vi "Write SP Operation Parameters.vi"(8 "error in (no error)":errorcluster, 10 "SP Operation Parameters":T1={"SP Load Less Than Thr?"=TRUE, "SP Load Threshold (um)"=4800.0, "SP Current Location"={"X (um)"=20.0, "Y (um)"=20.0, "Z (um)"=20.0, "T (degree)"=20.0}, "SP Chuck Speeds"={"XY Speed (10-100%)"=10.0, "Z Speed (10-100%)"=10.0, "T Speed (10-100%)"=10.0}, "Manual Step Parameters"={"Step in X"=FALSE, "X S-Speed [µm/step]"=5.0, "Step in Y"=FALSE, "Y S-Speed [µm/step]"=5.0, "Step in Z"=FALSE, "Z S-Speed [µm/step]"=5.0, "Step in T"=FALSE, "T S-Speed [mdegree/step]"=5.0, "X Increase"=TRUE, "Y Increase?"=TRUE, "Z Increase?"=TRUE, "T Increase?"=TRUE}, "Z Stepper"={"UP/DOWN"=FALSE, "UP/DOWN Speed [µm/step]"=20, "SP Z Step"=FALSE}, "Z Heights Set"=FALSE, "SP Contact Search"={"Contact Circuit"=enum."1", "Speed [1000-10000]"=1000.0, "Start Height [µm]"=0.0, "Search Band [µm]"=100.0, "Overdrive [µm]"=30.0}, "Separation Distance [µm]"=0, "Contact Height [µm]"=0, "Use Overdrive?"=FALSE, "Touchdown method"=enum."no feedback", "Arduino Edgesense params"={"touchdown height [µm]"=0, "search band [µm]"=100, "speed [µm/step]"=10, "overdrive [µm]"=30}} {"SP Contact Search"."Speed [1000-10000]" min=1000 max=10000; "SP Load Threshold (um)" format="%#_6f"}, 11 "SemiProbe in":refnum<class "SemiProbe.lvclass">) -> (0 "error out":errorcluster, 3 "SemiProbe out":refnum<class "SemiProbe.lvclass">)   [LabVIEW 2018, in "SemiProbe.lvclass"]
uses:
  SemiProbe.lvclass
  SemiProbe.lvclass/SemiProbe.ctl
panel:
  # "Of value set in the SP Navigation panel."
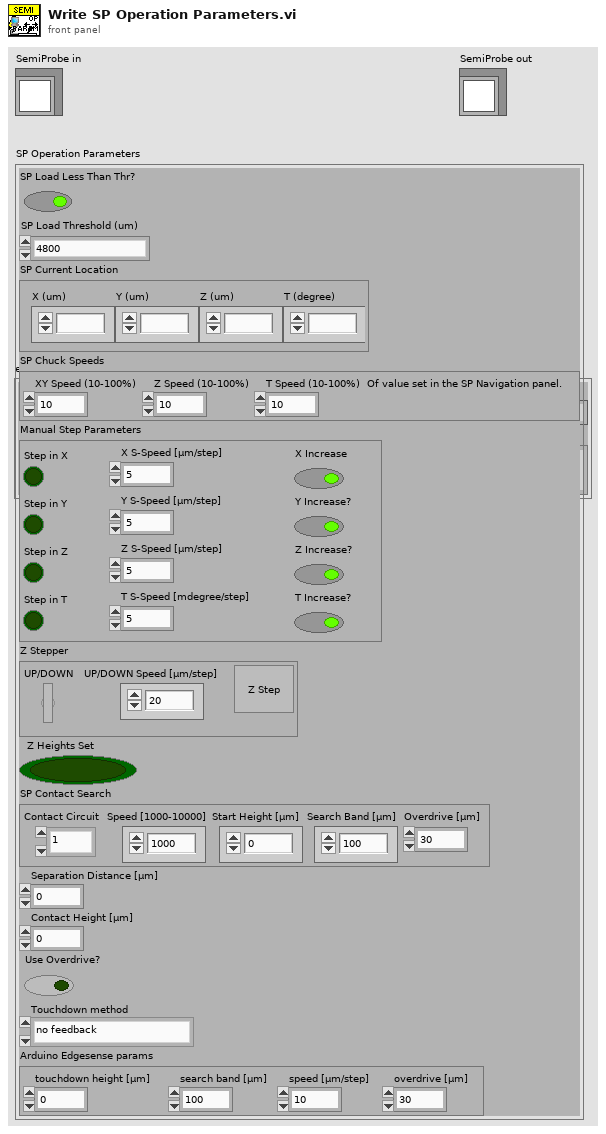
[diagram p1: front panel]
types:
  T1 = cluster{"SP Load Less Than Thr?":bool, "SP Load Threshold (um)":dbl, "SP Current Location":cluster{"X (um)":ext, "Y (um)":ext, "Z (um)":ext, "T (degree)":ext}, "SP Chuck Speeds":cluster{"XY Speed (10-100%)":dbl, "Z Speed (10-100%)":dbl, "T Speed (10-100%)":dbl}, "Manual Step Parameters":cluster{"Step in X":bool, "X S-Speed [µm/step]":sgl, "Step in Y":bool, "Y S-Speed [µm/step]":sgl, "Step in Z":bool, "Z S-Speed [µm/step]":sgl, "Step in T":bool, "T S-Speed [mdegree/step]":sgl, "X Increase":bool, "Y Increase?":bool, "Z Increase?":bool, "T Increase?":bool}, "Z Stepper":cluster{"UP/DOWN":bool, "UP/DOWN Speed [µm/step]":i32, "SP Z Step":bool}, "Z Heights Set":bool, "SP Contact Search":cluster{"Contact Circuit":enum16{"12", "1", "2"}, "Speed [1000-10000]":sgl, "Start Height [µm]":sgl, "Search Band [µm]":sgl, "Overdrive [µm]":sgl}, "Separation Distance [µm]":u32, "Contact Height [µm]":u32, "Use Overdrive?":bool, "Touchdown method":enum16{"no feedback", "Arduino edgesense", "SP contact circuit"}, "Arduino Edgesense params":cluster{"touchdown height [µm]":i32, "search band [µm]":u32, "speed [µm/step]":u32, "overdrive [µm]":u32}}
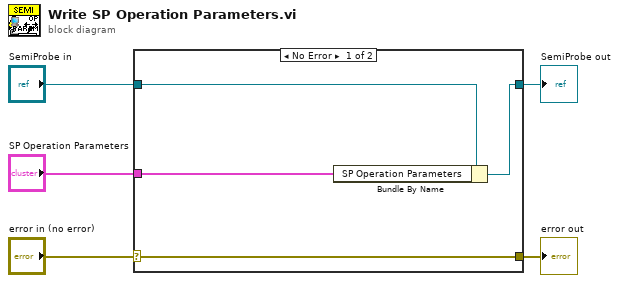
[diagram p0: block diagram]
diagram:
  n1 = case shown="No Error" "error in (no error)" {
    selector: "error in (no error)" -> [w9 w10]
    tunnel: [w9 w10] -> w4
    tunnel: [w7 w11] -> w2
    tunnel: "SemiProbe in" -> [w8 w11]
    tunnel: "SP Operation Parameters" -> [w6 _]
    frame No Error {
      n2 = Bundle By Name(cluster=w8, "SP Operation Parameters"=w6) -> (w7:refnum<class "SemiProbe.lvclass">)
    }
    frame Error {
    }
  }
  "error out" <- w4
  "SemiProbe out" <- w2
